vi "Load_Wine.vi"(8 "error in":errorcluster caption="entrée d'erreur") -> (0 "error out":errorcluster caption="sortie d'erreur", 3 "Tableau":string[][](array[string]))   [LabVIEW 2020]
doc: "Data Set Characteristics : \n\nNumber of Instances : 178 (50 in each of three classes)\n\nNumber of Attributes : 13 numeric, predictive attributes and the class\n\nAttribute Information : \n - Alcohol\n - Malic acid\n - Ash\n - Alcalinity of ash\n - Magnesium\n - Total phenols\n - Flavanoids\n - Nonflavanoid phenols\n - Proanthocyanins\n - Color intensity\n - Hue\n - OD280/OD315 of diluted wines\n - Proline\n\nclass :\n - class_0\n - class_1\n - class_2\n\nSummary Statistics : \n\n Alcohol : 11.0 14.8 13.0 0.8\n Malic Acid : 0.74 5.80 2.34 1.12\n Ash : 1.36 3.23 2.36 0.27\n Alcalinity of Ash : 10.6 30.0 19.5 3.3\n Magnesium : 70.0 162.0 99.7 14.3\n Total Phenols : 0.98 3.88 2.29 0.63\n Flavanoids : 0.34 5.08 2.03 1.00\n Nonflavanoid Phenols : 0.13 0.66 0.36 0.12\n Proanthocyanins : 0.41 3.58 1.59 0.57\n Colour Intensity : 1.3 13.0 5.1 2.3\n Hue : 0.48 1.71 0.96 0.23\n OD280/OD315 of diluted wines: 1.27 4.00 2.61 0.71\n Proline : 278 1680 746 315\n\nMissing Attribute Values : None\n\nClass Distribution : \n - class_0 (59)\n - class_1 (71)\n - class_2 (48)\n\nCreator : R.A. Fisher\n\nDonor : Michael Marshall (MARSHALL%PLU@io.arc.nasa.gov)\n\nDate : July, 1988\n\nThis is a copy of UCI ML Wine recognition datasets : https://archive.ics.uci.edu/ml/machine-learning-databases/wine/wine.data\n\nThe data is the results of a chemical analysis of wines grown in the same region in Italy by three different cultivators. There are thirteen different measurements taken for different constituents found in the three types of wine.\n\nOriginal Owners :\n\nForina, M. et al, PARVUS - An Extendible Package for Data Exploration, Classification and Correlation. Institute of Pharmaceutical and Food Analysis and Technologies, Via Brigata Salerno, 16147 Genoa, Italy."
uses:
  Load_Wine.lvclass
panel:
  out "Load_Wine en sortie":refnum<class "Load_Wine.lvclass">
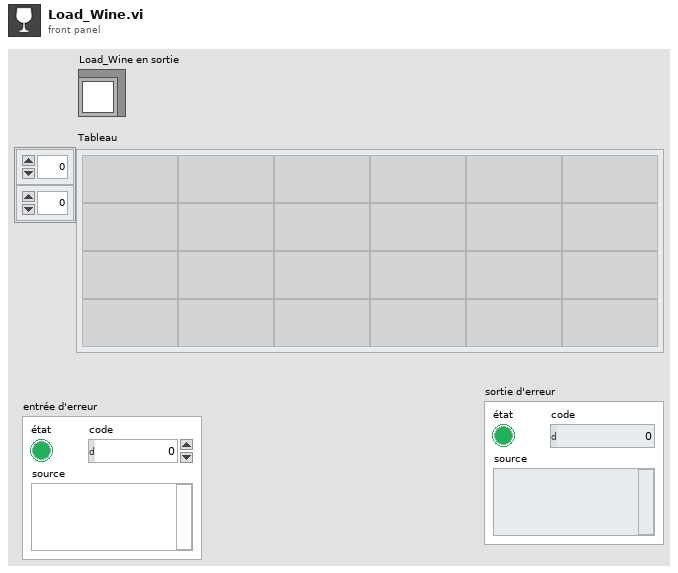
[diagram p1: front panel]
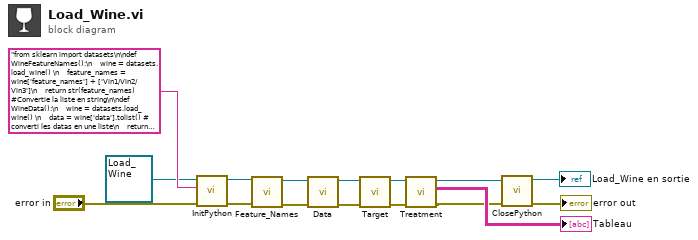
[diagram p0: block diagram]
diagram:
  n1 = call-dynamic "InitPython.vi"("error in (no error)"="error in", "Python Instruction"="from sklearn import datasets\n\ndef WineFeatureNames():\n    wine = datasets.load_wine() \n    feature_names = wine['feature_names'] + ['Vin1/Vin2/Vin3']\n    return str(feature_names) #Convertie la liste en string\n\ndef WineData():\n    wine = datasets.load_wine() \n    data = wine['data'].tolist() # converti les datas en une liste\n    return str(data) #Convertie la liste en string\n\ndef WineTarget():\n    wine = datasets.load_wine() \n    data_target = wine['target'].tolist() # converti les datas en une liste\n    return str(data_target) #Convertie la liste en string\n", "Scikit-learn en entrée"=refnum<class "Load_Wine.lvclass"> refnum ("Load_Wine.lvclass")) -> ("error out"=w11:errorcluster, "Scikit-learn en sortie"=w12:refnum<class "Load_Wine.lvclass">)  [unwired: 7 in]
  n2 = call-dynamic "Feature_Names.vi"("error in (no error)"=w11, "Load_Wine en entrée"=w12) -> ("error out"=w9:errorcluster, "Load_Wine en sortie"=w10:refnum<class "Load_Wine.lvclass">)  [unwired: 8 in]
  n3 = call-dynamic "Data.vi"("error in (no error)"=w9, "Load_Wine en entrée"=w10) -> ("error out"=w7:errorcluster, "Load_Wine en sortie"=w8:refnum<class "Load_Wine.lvclass">)  [unwired: 8 in]
  n4 = call-dynamic "Target.vi"("error in (no error)"=w7, "Load_Wine en entrée"=w8) -> ("error out"=w5:errorcluster, "Load_Wine en sortie"=w6:refnum<class "Load_Wine.lvclass">)  [unwired: 8 in]
  n5 = call-dynamic "Treatment.vi"("error in (no error)"=w5, "Load_Wine en entrée"=w6) -> ("error out"=w2:errorcluster, "Tableau"=→"Tableau":string[][], "Load_Wine en sortie"=w4:refnum<class "Load_Wine.lvclass">)  [unwired: 7 in]
  n6 = call-dynamic "ClosePython.vi"("error in (no error)"=w2, "Scikit-learn en entrée"=w4) -> ("error out"=→"error out":errorcluster, "Scikit-learn en sortie"=→"Load_Wine en sortie":refnum<class "Load_Wine.lvclass">)  [unwired: 8 in]
